vi "MyGlobal.vi"() -> ()   [LabVIEW 2020]
panel:
  in  "right trigger":sgl
  in  "left trigger":sgl
  in  "POV":sgl
  in  "Bouton arriere gauche":bool
  in  "Bouton arriere droit":bool
  in  "Bouton Y":bool
  in  "Bouton X":bool
  in  "Bouton B":bool
  in  "Bouton A":bool
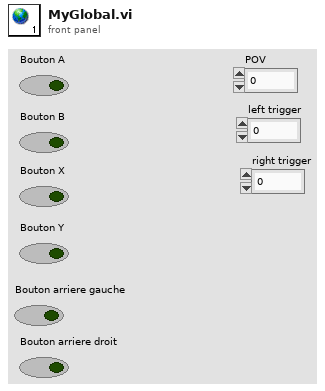
[diagram p1: front panel]
diagram:
